vi "State History.vi"(7 "State":string) -> (5 "State History":string)   [LabVIEW 2019, in "Database Viewer.lvclass"]
uses:
  Database Viewer.lvclass
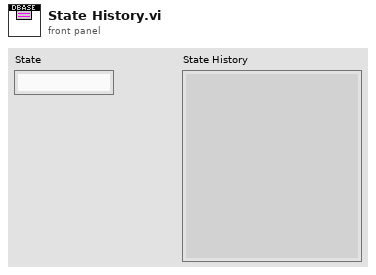
[diagram p1: front panel]
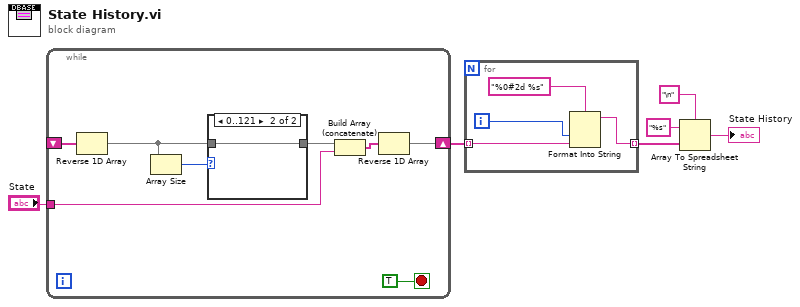
[diagram p0: block diagram]
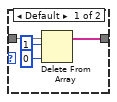
[diagram p2: hidden frame]
diagram:
  n1 = while {
    shift-right: [w7] -> w2
    shift-left: _ -> [w13]
    tunnel: "State" -> [w9]
    stop <- TRUE stop-if-true
    n2 = Reverse 1D Array(array=w13) -> (reversed array=w8:string[])
    n3 = Array Size(array=w8) -> (size(s)=w12:i32)
    n4 = case shown="0..121" w12 {
      tunnel: [w17 w19] -> w11
      tunnel: w8 -> [w18 w19]
      frame Default {
        n5 = Delete From Array(array=w18, length=1, index=0) -> (array with subset deleted=w17:string[])  [unwired: 1 out]
      }
      frame 0..121 {
      }
    }
    n6 = Build Array (concatenate)(w11, w9) -> (w10:string[])
    n7 = Reverse 1D Array(array=w10) -> (reversed array=w7:string[])
  }
  n8 = for {
    tunnel: w2 -> [w22] mode=indexing
    tunnel: [w20] -> w1 mode=indexing
    i -> [w21]
    n9 = Format Into String(format string="%0#2d %s", w21, w22) -> (resulting string=w20:string)  [unwired: 2 in, 1 out]
  }
  n10 = Array To Spreadsheet String(delimiter (Tab)="\n", array=w1, 3:"%s" ("format string")) -> (spreadsheet string=→"State History":string)
